vi "RFH-convert-libreVNA.vi"(5 "destionation path":path, 7 "All libreVNA data folder":path) -> (0 "error out":errorcluster, 2 "last file":path)   [LabVIEW 2020, in "RFH-Reflection_File_Handler.lvlib"]
uses:
  RFH-Reflection_File_Handler.lvlib
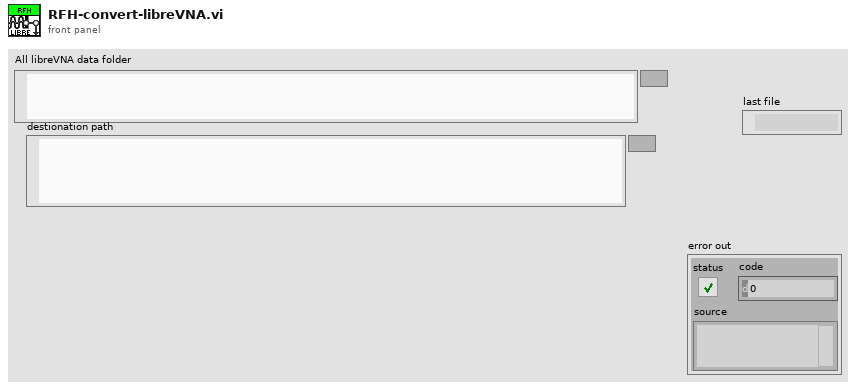
[diagram p1: front panel]
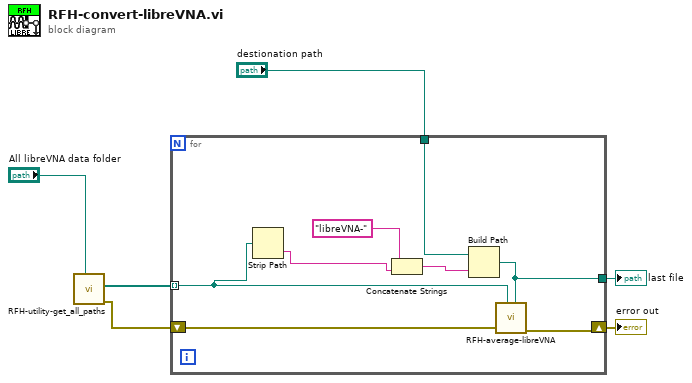
[diagram p0: block diagram]
diagram:
  n1 = call "RFH-utility-get_all_paths.vi"("Folder Path"="All libreVNA data folder") -> ("error out"=w3:errorcluster, "All Folders"=w5:path[])  [unwired: 7 in, 2 out]
  n2 = for {
    tunnel: w5 -> [w12] mode=indexing
    tunnel: "destionation path" -> [w10]
    shift-right: [w8] -> w2
    shift-left: w3 -> [w9]
    tunnel: [w7] -> w1
    n3 = Strip Path(path=w12) -> (name=w11:string)  [unwired: 1 out]
    n4 = Concatenate Strings("libreVNA-" ("string"), w11) -> (w14:string)
    n5 = Build Path(base path=w10, name or relative path=w14) -> (appended path=w7:path)
    n6 = call "RFH-average-libreVNA.vi"("average filepath"=w7, "Source Folder"=w12, "error in (no error)"=w9) -> ("error out"=w8:errorcluster)  [unwired: 8 in]
  }
  "error out" <- w2
  "last file" <- w1
